vi "GetAlazar_SynthFoc.vi"(0 "AlazarCluster":T8, 1 "Digitizer Settings":T4={"Digitizer delay (us) "=0.0, "rf points per line"=2048, "lines per plane"=128, "Samp Rate (Hz)"=100000000.0, "Additional dig delay (us)"=0.0, "Voltage Scale"=0.4, "Pre-Looks"=0, "Offset delay (us)"=0.0, "bits A/D"=8, "Avg Num"=1, "DigTimeOut"=5.0, "Rel Dig Delay"=0.0, "Dig Ch"=0, "LeCroyCluster"={"LeCroy Channels"=[TRUE, FALSE, FALSE, FALSE], "LC read pt offset"=0.0, "Sweep Avg"=FALSE}, "Main Digitizer"=enum."NI Digitizer", "Dig Config"=enum."Single channel", "Digitizer ID Cluster"={"Acqiris/Alazar/SP ID"=[], "NI Instr Handles"=[], "LeCroy VISA"="", "GaGe Handle"={"Handle"=0, "Sample size"=0, "Resolution"=0, "Offset"=0, "Channels"=0, "Boards"=0}, "ATS Ref"="ATS9350", "Acqiris Address"=["PCI::INSTR0"], "ADQRef"=refnum, "adq_cu_ptr"=refnum}, "Trigger Settings"={"Trig Source"=1, "Trig Coupling"=0, "Trig Slope"=0, "Level (mV)"=1500.0}, "Bulk Acq"=FALSE, "Bulk Start Indexes"=[], "Data Ref RF"=refnum, "NI ID/Channel"=[], "Total Dig CH"=1, "Xtra Ann Trig delay (us)"=10.0, "Fix Z Delay?"=FALSE, "One Way Transmission?"=FALSE, "Data Ref Log"=refnum} {"Trigger Settings"."Trig Slope" items=["Positive", "Negative"]; "Trigger Settings"."Level (mV)" format="%.2f"; "Trigger Settings"."Trig Coupling" items=["DC 1 MOhm", "AC 1 MOhm", "DC 50 Ohm", "AC 50 Ohm"]; "Trigger Settings"."Trig Source" items=["Chan 1", "External"]; "Rel Dig Delay" format="%.2f"; "DigTimeOut" format="%.2f"; "Avg Num" min=1; "Offset delay (us)" format="%.2f"; "Additional dig delay (us)" format="%.2f"; "Digitizer delay (us)" format="%.2f"}, 7 "errorin":errorcluster, 8 "File Array":string[](array[string]), 9 "Ann Array Params":T1={"Synth Foc?"=FALSE, "Focal Zones"=41, "Switch T/R"=0, "Trans Geometry (mm)"={"Transducer"=0, "Geo Focus"=12.0, "a (radius)"=3.0, "# of rings"=5, "kerf space "=0.1, "Center Freq"=12.0}, "Sub Ap Excite?"=FALSE, "Full Array Scan?"=FALSE, "Xmt/Rcv"={"XMIT"=[TRUE, TRUE, TRUE, TRUE, TRUE], "RCV"=[TRUE, TRUE, TRUE, TRUE, TRUE]}, "PulseSpacing (us)"=0.0, "Xmit Ring"=0, "XMIT CHS"=0, "RCV CHS"=0, "GPU?"=FALSE, "Save TIFF?"=FALSE, "downfactor"=1, "RCV 1CH"=0} {"RCV 1CH" items=["All", "1", "2", "3", "4", "5"]; "Trans Geometry (mm)"."Transducer" items=["6D 12R 40 MHz"=0, "10D 31R 20 MHz"=1, "10D 23R 20 MHz"=2, "6D 23R 40 MHz"=3, "4.5D 10.7R 40 MHz"=4, "9D 23.5R 20 MHz"=5, "9D 25.8R 20MHz"=6, "Enter"=99]; "Switch T/R" min=1 max=5 step=1}, 10 "lines per plane":i32, 11 "Reverse ?":bool, 13 "Rcv Ring":i32) -> (17 "Raw VGain (scale)":dbl, 18 "Gain Array":T10(array[cluster]), 21 "VGain (dB)":dbl, 25 "Array out":i16[][][](array[numeric]), 27 "error out":errorcluster)   [LabVIEW 2022 SP3]
uses:
  Annular Array/-SynthApperture/ProcImageHD_I16.vi
  -DigitizerRoutines/DigitizerSettings.ctl
  -DigitizerRoutines/DigitizerID.ctl
  -DigitizerRoutines/Digitizer.ctl
  Annular Array/-AnnularRoutines/ArrayGeometry.ctl
  Annular Array/-AnnularRoutines/TransGeometry.ctl
  Annular Array/-AnnularRoutines/AnnularArray.ctl
  -DigitizerRoutines/DigConfig.ctl
  C:/Windows/System32/ADQAPI_dotNet_helper.dll
panel:
  out "Voltage Scale":T9
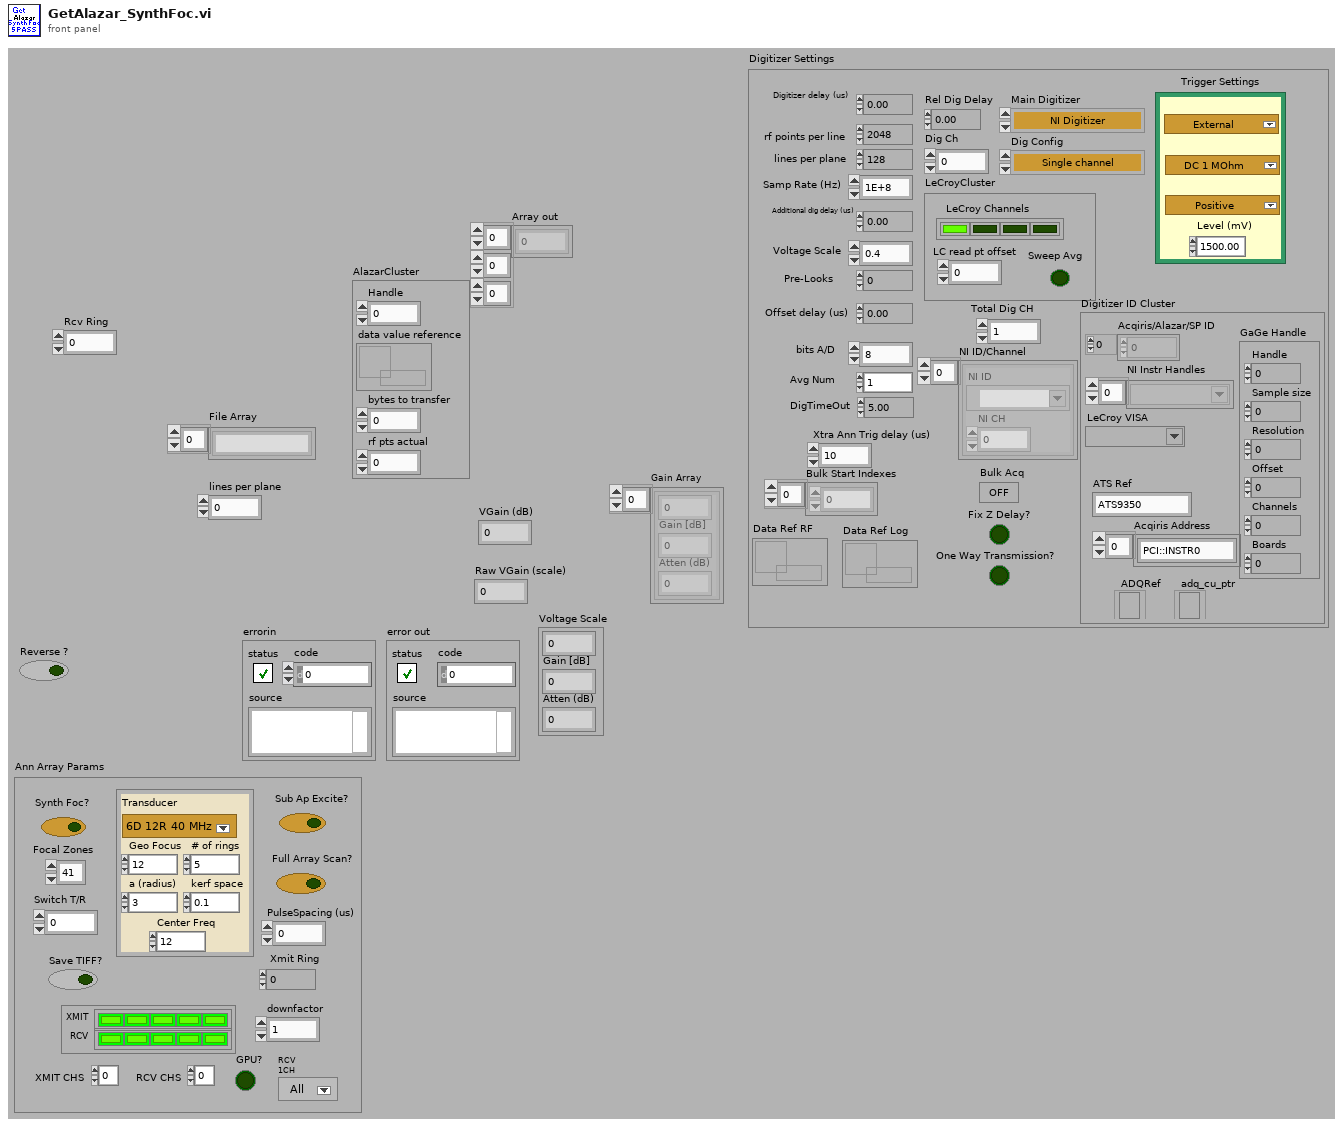
[diagram p1: front panel]
types:
  T1 = typedef "AnnularArray.ctl" = cluster{"Synth Foc?":bool, "Focal Zones":i16, "Switch T/R":i16, "Trans Geometry (mm)":T2, "Sub Ap Excite?":bool, "Full Array Scan?":bool, "Xmt/Rcv":cluster{"XMIT":bool[], "RCV":bool[]}, "PulseSpacing (us)":sgl, "Xmit Ring":i32, "XMIT CHS":u8, "RCV CHS":u8, "GPU?":bool, "Save TIFF?":bool, "downfactor":i32, "RCV 1CH":u16}
  T2 = typedef "TransGeometry.ctl" = cluster{"Transducer":T3, "Geo Focus":dbl, "a (radius)":dbl, "# of rings":i32, "kerf space ":dbl, "Center Freq":dbl}
  T3 = typedef "ArrayGeometry.ctl" = u16
  T4 = typedef "DigitizerSettings.ctl" = cluster{"Digitizer delay (us) ":dbl, "rf points per line":i32, "lines per plane":i32, "Samp Rate (Hz)":dbl, "Additional dig delay (us)":dbl, "Voltage Scale":dbl, "Pre-Looks":i32, "Offset delay (us)":dbl, "bits A/D":i8, "Avg Num":i32, "DigTimeOut":sgl, "Rel Dig Delay":sgl, "Dig Ch":i32, "LeCroyCluster":cluster{"LeCroy Channels":bool[], "LC read pt offset":dbl, "Sweep Avg":bool}, "Main Digitizer":T5, "Dig Config":T6, "Digitizer ID Cluster":T7, "Trigger Settings":cluster{"Trig Source":u16, "Trig Coupling":u16, "Trig Slope":u16, "Level (mV)":dbl}, "Bulk Acq":bool, "Bulk Start Indexes":i32[], "Data Ref RF":refnum<data-value>, "NI ID/Channel":cluster{"NI ID":refnum<k15>, "NI CH":i32}[], "Total Dig CH":i32, "Xtra Ann Trig delay (us)":dbl, "Fix Z Delay?":bool, "One Way Transmission?":bool, "Data Ref Log":refnum<data-value>}
  T5 = typedef "Digitizer.ctl" = enum16{"Acqiris Digitizer", "NI Digitizer", "LeCroy", "GaGe", "AlazarTech", "No Digitizer", "Teledyne"}
  T6 = typedef "DigConfig.ctl" = enum16{"Single channel", "2 Chans w/ 2 Acqiris", "2 Chans w/ 1 Acqiris", "5-CH Pulser New", "5-CH pulser w/ ann array", "5-pass style ann array", "Empty"}
  T7 = typedef "DigitizerID.ctl" = cluster{"Acqiris/Alazar/SP ID":u32[], "NI Instr Handles":refnum<k15>[], "LeCroy VISA":refnum<visa-resource-name>, "GaGe Handle":cluster{"Handle":u32, "Sample size":u32, "Resolution":i32, "Offset":i32, "Channels":u32, "Boards":u32}, "ATS Ref":string, "Acqiris Address":string[], "ADQRef":refnum<k24>, "adq_cu_ptr":refnum<k24>}
  T8 = cluster{"Handle":u32, "data value reference":refnum<data-value>, "bytes to transfer":u32, "rf pts actual":u32}
  T9 = cluster{sgl, "Gain [dB]  ":sgl, "Atten (dB)":sgl}
  T10 = cluster{sgl, "Gain [dB]  ":sgl, "Atten (dB)":sgl}[]
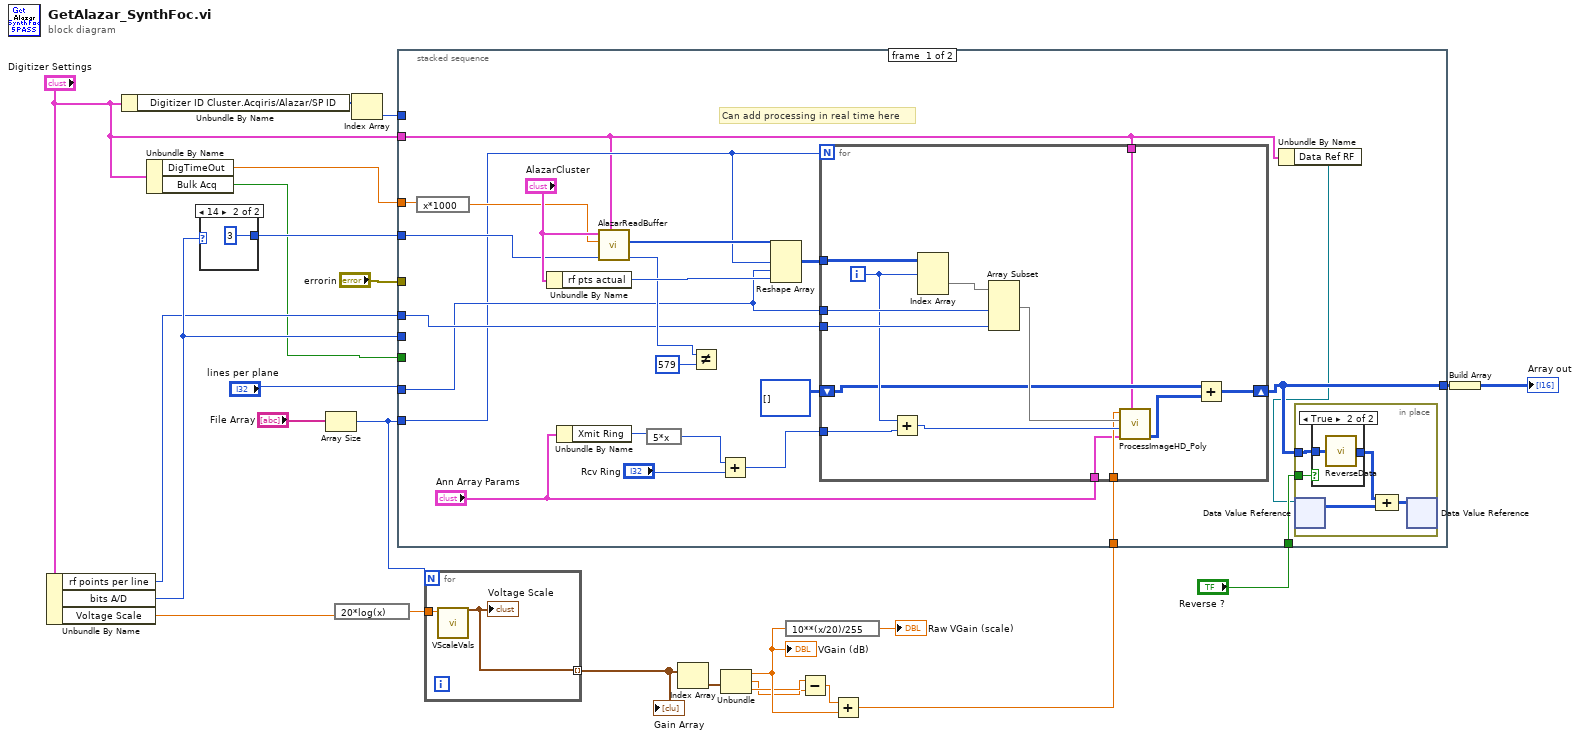
[diagram p0: block diagram]
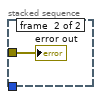
[diagram p4: hidden frame]
diagram:
  n1 = Unbundle By Name("Digitizer Settings") -> ("rf points per line"=w5:i32, "bits A/D"=w6:i8, "Voltage Scale"=w7:dbl)
  n2 = Unbundle By Name("Digitizer Settings") -> ("Digitizer ID Cluster.Acqiris/Alazar/SP ID"=w22:u32[])
  n3 = Unbundle By Name("Digitizer Settings") -> ("DigTimeOut"=w4:sgl, "Bulk Acq"=w3:bool)
  n4 = case shown="14" w6 {
    tunnel: [_ u16 3 ("Extra Shift")] -> w20
    frame 0, Default {
    }
    frame 14 {
    }
  }
  n5 = Array Size(array="File Array") -> (size(s)=w15:i32)
  n6 = expression code="20*log(x)"(w7) -> (w16:dbl)
  n7 = Index Array(array=w22) -> (element=w21:u32)  [unwired: 1 in]
  n8 = for {
    N: w15 -> [_]
    tunnel: [w27] -> w19 mode=indexing
    tunnel: w16 -> [w28]
    n9 = call "VScaleVals.vi"("Full Scale"=w28) -> ("Voltage Scale"=w27:T9)  [unwired: 8 in, 2 out]
    "Voltage Scale" <- w27
  }
  "Gain Array" <- w19
  n10 = Index Array(array=w19) -> (element=w17:T9)  [unwired: 1 in]
  n11 = Unbundle(w17) -> (w13:sgl, "Gain [dB]"=w11:sgl, "Atten (dB)"=w12:sgl)
  "VGain (dB)" <- w13
  n12 = expression code="10**(x/20)/255"(w13) -> (→"Raw VGain (scale)":sgl)
  n13 = Subtract(x=w12, y=w11) -> (x-y=w14:sgl)
  n14 = Add(x=w14, y=w13) -> (x+y=w10:sgl)
  n15 = stacked-sequence {
    tunnel: w4 -> [w43 _]
    tunnel: "lines per plane" -> [w44 _]
    tunnel: w5 -> [w45 _]
    tunnel: "errorin" -> [_ w74]
    tunnel: w15 -> [w40 _]
    tunnel: w6 -> [_ _]
    tunnel: w3 -> [_ _]
    tunnel: w21 -> [_ _]
    tunnel: w20 -> [w41 _]
    tunnel: w10 -> [w36 _]
    tunnel: [w32 _] -> w9
    tunnel: "Digitizer Settings" -> [w30 _]
    tunnel: "Reverse ?" -> [w31 _]
    frame #0 {
      # "Can add processing in real time here"
      n16 = expression code="x*1000"(w43) -> (w42:sgl)
      n17 = Unbundle By Name("AlazarCluster") -> ("rf pts actual"=w49:u32)
      n18 = Unbundle By Name("Ann Array Params") -> ("Xmit Ring"=w34:i32)
      n19 = call "AlazarReadBuffer.vi"("Digitizer Settings"=w30, "Extra Shift"=w41, "time out"=w42, "AlazarCluster"="AlazarCluster") -> ("Return Code"=w48:u32, "Data Array"=w50:i16[])  [unwired: 5 in, 1 out]
      n20 = expression code="5*x"(w34) -> (w39:i32)
      n21 = Not Equal?(x=w48, y=u32 579) -> ()  [unwired: 1 out]
      n22 = Add(x=w39, y="Rcv Ring") -> (x+y=w37:i32)
      n23 = Reshape Array(w50, w40, w44, w49) -> (w51:i16[][][])
      n24 = for {
        N: w40 -> [_]
        tunnel: w51 -> [w73]
        tunnel: w45 -> [w72]
        tunnel: w44 -> [w71]
        tunnel: w37 -> [w68]
        tunnel: w36 -> [w65]
        shift-right: [w63] -> w32
        shift-left: i16[][] [] -> [w62]
        tunnel: w30 -> [w61]
        tunnel: "Ann Array Params" -> [w60]
        i -> [w69]
        n25 = Add(x=w69, y=w68) -> (x+y=w67:i32)
        n26 = Index Array(array=w73, index (dim 0)=w69) -> (element=w70:i16[][])  [unwired: 2 in]
        n27 = Array Subset(array=w70, length (row)=w71, length (col)=w72) -> (w66:i16[][])  [unwired: 2 in]
        n28 = call-poly "ProcessImageHD_Poly.vi"("Digitizer Settings"=w61, "Ann Array Params"=w60, "T/R Ring"=w67, "Scan Data In"=w66, "Att (dB)"=w65) -> ("Synth App Out"=w64:i16[][])  [unwired: 3 in, 1 out]
        n29 = Add(x=w62, y=w64) -> (x+y=w63:i16[][])
      }
      n30 = Unbundle By Name(w30) -> ("Data Ref RF"=w29:refnum<data-value>)
      n31 = in-place {
        in-place-border: w32 -> [w53]
        in-place-border: w31 -> [w52]
        n32 = in-place-dvr #1(w29) -> (w56:i16[][])  [unwired: 1 out]
        n33 = case shown="True" w52 {
          tunnel: w53 -> [w57 w59]
          tunnel: [w57 w58] -> w54
          frame False {
          }
          frame True {
            n34 = call "ReverseData.vi"("Array in"=w59) -> ("Array out"=w58:i16[][])
          }
        }
        n35 = Compound Arithmetic op=ADD(w54, w56) -> (w55:i16[][])
        n36 = in-place-dvr #1(w55) -> ()  [unwired: 2 out]
      }
    }
    frame #1 {
      "error out" <- w74
    }
  }
  n37 = Build Array(w9) -> (→"Array out":i16[][][])
